vi "TimestampToSecondsSince.vi"(1 "Time Stamp Control":timestamp=timestamp(3428950268.958698 s since 1904-01-01) format="%<%H:%M\n%d-%b-%Y>T") -> (0 "unsigned 32bit integer":u32 caption="SecondsSince1Jan1904")   [LabVIEW 2011]
panel:
  out "unsigned 64bit integer":u64
  out "double precision float":dbl format="%#.6f"
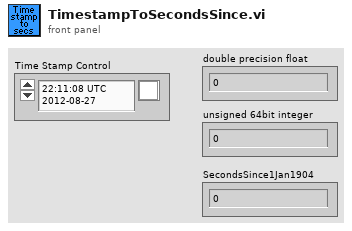
[diagram p1: front panel]
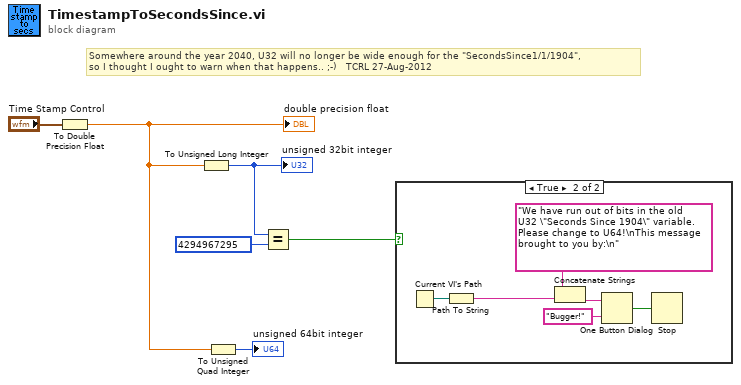
[diagram p0: block diagram]
diagram:
  # "Somewhere around the year 2040, U32 will no longer be wide enough for the \"SecondsSince1/1/1904\",\nso I thought I ought to warn when that happens.. ;-)   TCRL 27-Aug-2012"
  n1 = To Double Precision Float(number="Time Stamp Control") -> (double precision float=w2:dbl)
  "double precision float" <- w2
  n2 = To Unsigned Long Integer(number=w2) -> (unsigned 32bit integer=w5:u32)
  "unsigned 32bit integer" <- w5
  n3 = To Unsigned Quad Integer(1:w2) -> (0:→"unsigned 64bit integer":u64)
  n4 = Equal?(x=w5, y=u32 4294967295) -> (x = y?=w3:bool)
  n5 = case shown="True" w3 {
    frame False {
    }
    frame True {
      n6 = Current VI's Path() -> (path=w8:path)
      n7 = Path To String(path=w8) -> (string=w7:string)
      n8 = Concatenate Strings("We have run out of bits in the old U32 \"Seconds Since 1904\" variable. Please change to U64!\nThis message brought to you by:\n" ("message"), w7) -> (w9:string)
      n9 = One Button Dialog(message=w9, button name ("OK")="Bugger!") -> (true=w10:bool)
      n10 = Stop(stop? (T)=w10) -> ()
    }
  }
